vi "Update All Values.vi"(8 "error in (no error)":errorcluster, 10 "Values":refnum<class "Type.lvclass">[](array[class]), 11 "Game in":refnum<class "Game.lvclass">) -> (0 "error out":errorcluster, 3 "Game out":refnum<class "Game.lvclass">)   [LabVIEW 2022 SP3, in "Conditum-Example.lvlib" / "Game.lvclass"]
uses:
  Game.lvclass
  Conditum/Columns/Type/Type.lvclass
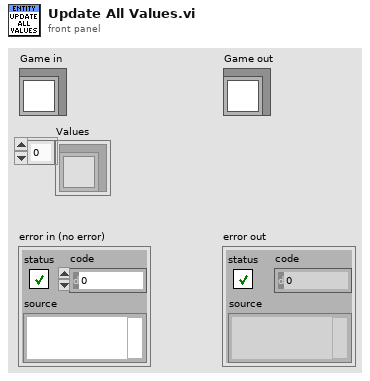
[diagram p1: front panel]
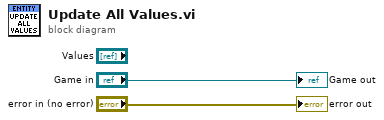
[diagram p0: block diagram]
diagram:
  "error out" <- "error in (no error)"
  "Game out" <- "Game in"
